vi "Calcul centroid.vi"(7 "Data PID":refnum<queue>, 8 "error in (no error)":errorcluster caption="entrée d'erreur (pas d'erreur)", 9 "Activer PID":bool, 10 "ROI":i16[][](array[numeric]), 11 "Data Cam Processing":T1 {"sigma X" format="%0.2f"; "mean X" format="%0.2f"; "mean Y" format="%0.2f"; "sigma Y" format="%0.2f"; "Shutter (us)" scale=22.0..10000000.0; "Gain Caméra" scale=0.0..1023.0}) -> (0 "error out":errorcluster caption="sortie d'erreur", 1 "CY brut":dbl, 2 "CX brut":dbl, 3 "Data Cam Processing 2":T1 {"sigma X" format="%0.2f"; "mean X" format="%0.2f"; "mean Y" format="%0.2f"; "sigma Y" format="%0.2f"; "Shutter (us)" scale=22.0..10000000.0; "Gain Caméra" scale=0.0..1023.0})   [LabVIEW 2026]
uses:
  Data-Processing.ctl
  <vilib>/Serenial/G Industrial Camera/g_industrial_cam/Buffer/Buffer.lvclass
  <vilib>/Serenial/G Industrial Camera/g_industrial_cam/Camera/Camera.lvclass
  <vilib>/picture/picture.llb/imagedata.ctl
  Data PID.ctl
  Etat_PID.ctl
  Set CX_CY.ctl
  <vilib>/ptbypt/NI_PtbyPt.lvlib
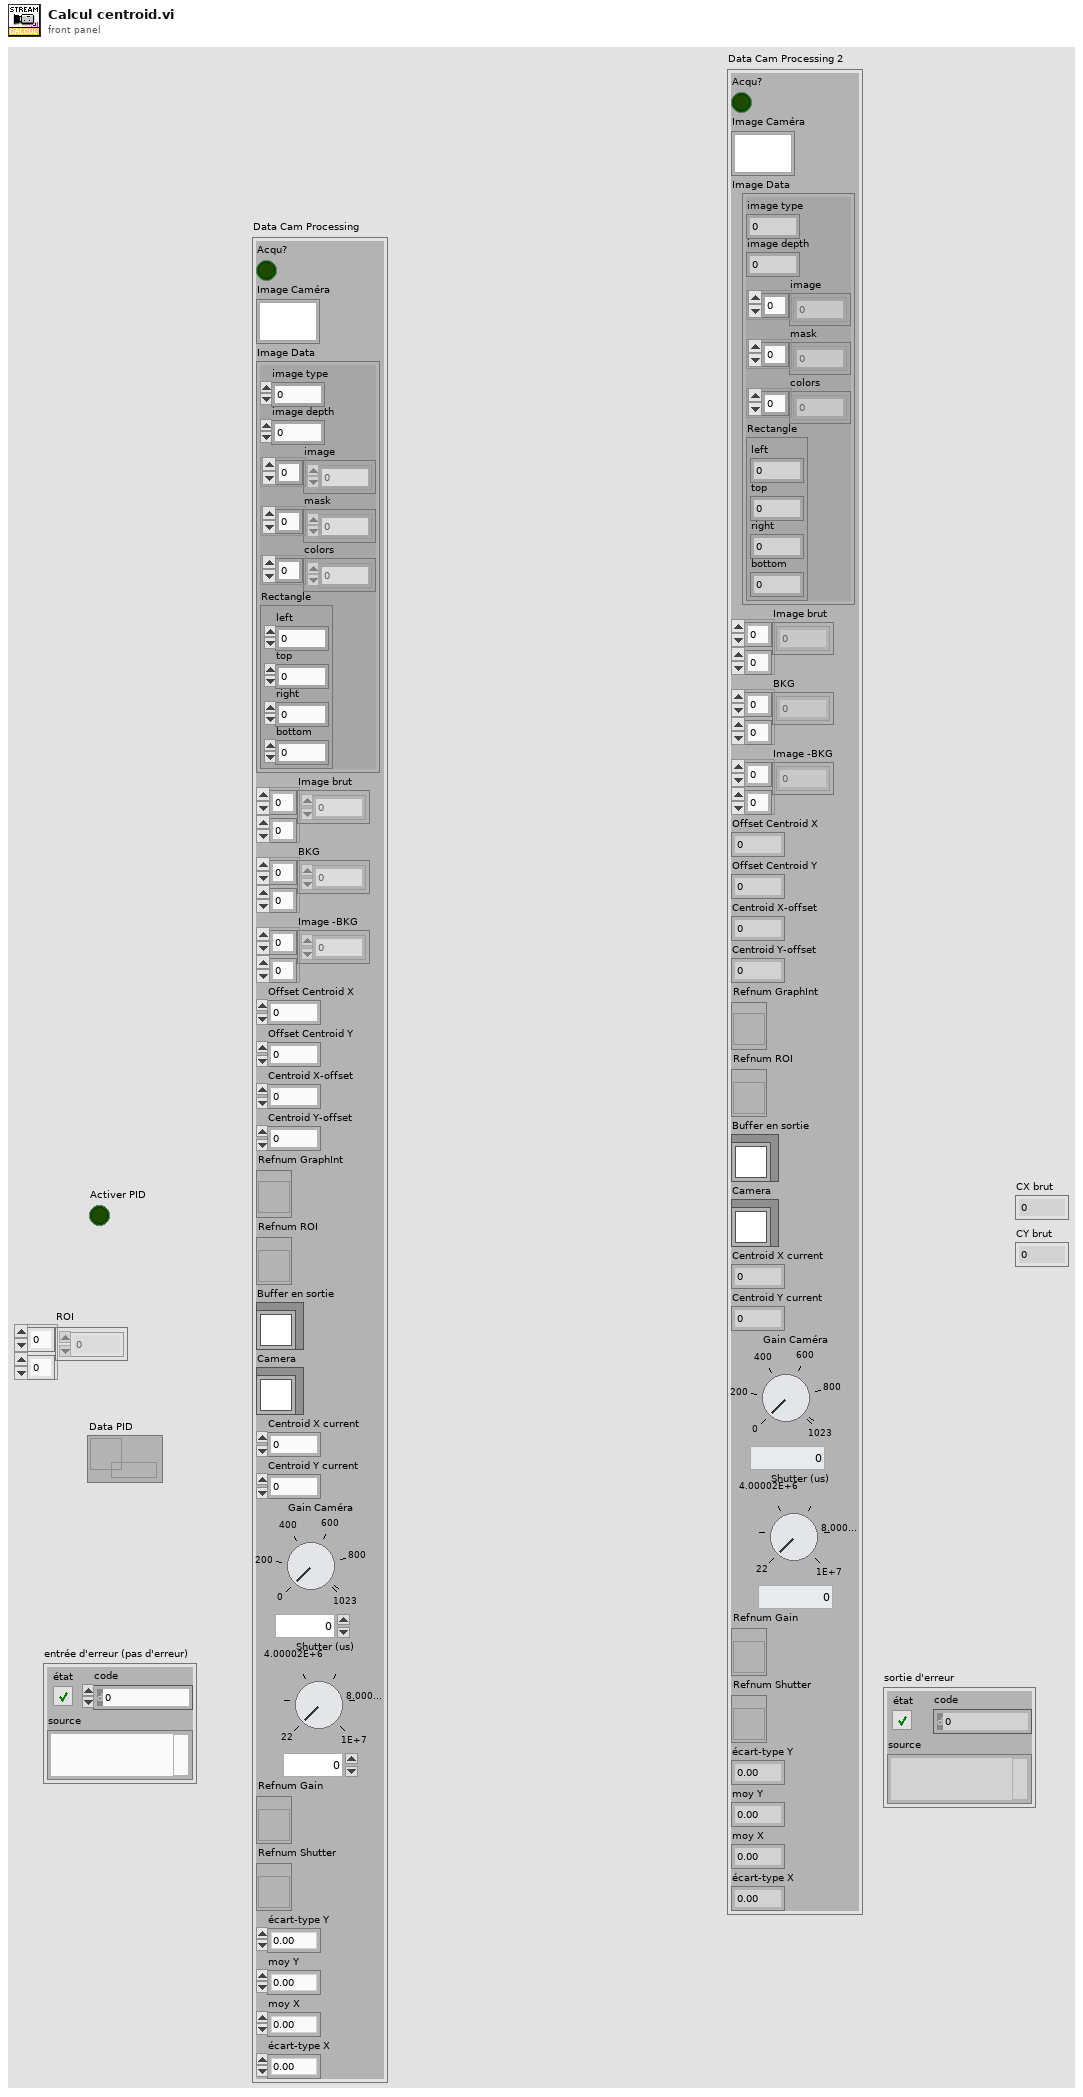
[diagram p1: front panel]
types:
  T1 = typedef "Data-Processing.ctl" = cluster{"Acqu?":bool, "Image Caméra":picture, "Image Data":T2, "Image brut":i16[][], "BKG":i16[][], "Image -BKG":i16[][], "Offset Centroid X":dbl, "Offset Centroid Y":dbl, "Centroid X-offset":dbl, "Centroid Y-offset":dbl, "Refnum GraphInt":refnum<vi>, "Refnum ROI":refnum<vi>, "Buffer en sortie":refnum<class "Buffer.lvclass">, "Camera":refnum<class "Camera.lvclass">, "Centroid X current":dbl, "Centroid Y current":dbl, "Gain Caméra":i32, "Shutter (us)":dbl, "Refnum Gain":refnum<vi>, "Refnum Shutter":refnum<vi>, "sigma Y":dbl, "mean Y":dbl, "mean X":dbl, "sigma X":dbl}
  T2 = typedef "imagedata.ctl" = cluster{"image type":i32, "image depth":i32, "image":u8[], "mask":u8[], "colors":u32[], "Rectangle":cluster{"left":i16, "top":i16, "right":i16, "bottom":i16}}
  T3 = typedef "Set CX_CY.ctl" = cluster{"CX":dbl, "CY":dbl}
  T4 = typedef "Etat_PID.ctl" = enum16{"PID", "Stop", "Reset PID", "Set Centroid", "Set T-Cube"}
  T5 = typedef "Data PID.ctl" = cluster{"Etat PID":T4, "Data PID":variant}
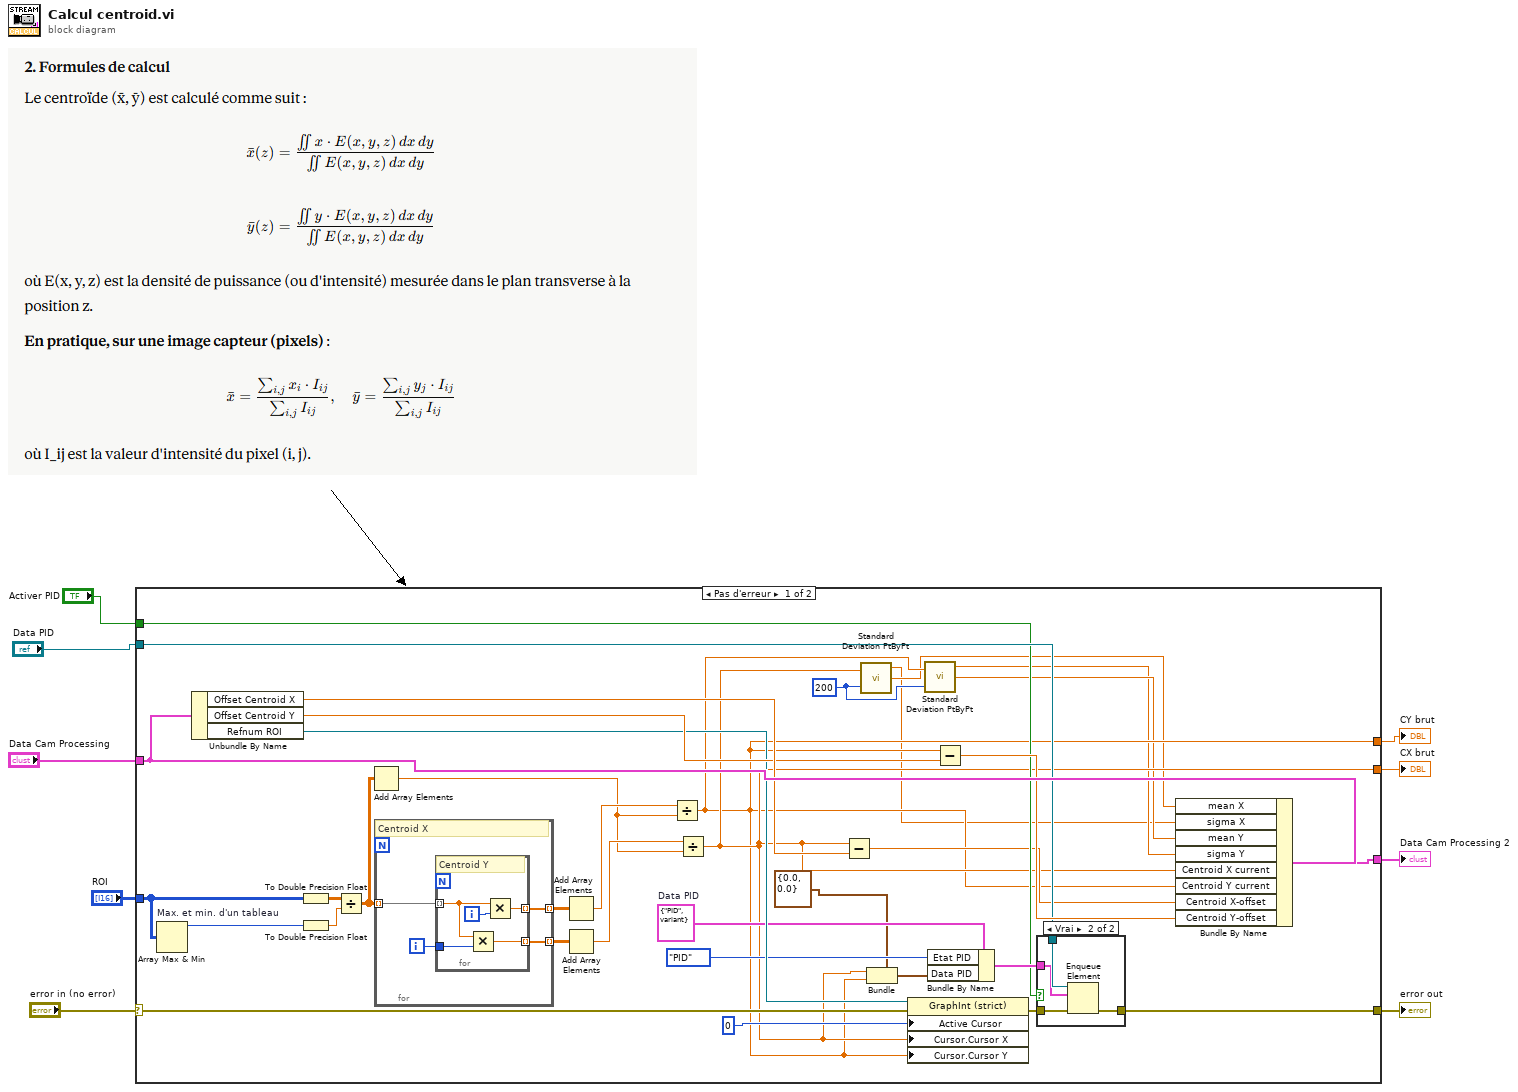
[diagram p0: block diagram]
diagram:
  n1 = case shown="Pas d'erreur" "error in (no error)" {
    selector: "error in (no error)" -> [w29 w60]
    tunnel: "ROI" -> [w38 _]
    tunnel: [w25 w60] -> w7
    tunnel: [w31 w59] -> w6
    tunnel: "Data Cam Processing" -> [w34 w59]
    tunnel: [w15 _] -> w4
    tunnel: [w14 _] -> w3
    tunnel: "Data PID" -> [w24 _]
    tunnel: "Activer PID" -> [w20 _]
    frame No Error {
      w16 = 200 ("sample length")
      w22 = T5 {"Etat PID"=enum."PID", "Data PID"=variant}  # Data PID
      n2 = Array Max & Min "Max. et min. d'un tableau"(array=w38) -> (max value=w39:i16)  [unwired: 3 out]
      n3 = Unbundle By Name(w34) -> ("Offset Centroid X"=w33:dbl, "Offset Centroid Y"=w32:dbl, "Refnum ROI"=w28:refnum<vi>)
      n4 = To Double Precision Float(number=w38) -> (double precision float=w36:dbl[][])
      n5 = To Double Precision Float(number=w39) -> (double precision float=w35:dbl)
      n6 = Divide(x=w36, y=w35) -> (x/y=w37:dbl[][])
      n7 = Add Array Elements(numeric array=w37) -> (sum=w40:dbl)
      n8 = for {
        tunnel: w37 -> [w52] mode=indexing
        tunnel: [w51] -> w44 mode=indexing
        tunnel: [w50] -> w42 mode=indexing
        i -> [w53]
        # "Centroid X"
        n9 = for {
          tunnel: w53 -> [w58]
          tunnel: w52 -> [w54] mode=indexing
          tunnel: [w57] -> w51 mode=indexing
          tunnel: [w55] -> w50 mode=indexing
          i -> [w56]
          # "Centroid Y"
          n10 = Multiply(x=w54, y=w58) -> (x*y=w57:dbl)
          n11 = Multiply(x=w54, y=w56) -> (x*y=w55:dbl)
        }
      }
      n12 = Add Array Elements(numeric array=w42) -> (sum=w41:dbl)
      n13 = Add Array Elements(numeric array=w44) -> (sum=w43:dbl)
      n14 = Divide(x=w41, y=w40) -> (x/y=w14:dbl)
      n15 = Divide(x=w43, y=w40) -> (x/y=w15:dbl)
      n16 = Subtract(x=w15, y=w33) -> (x-y=w19:dbl)
      n17 = call <vilib>:"Standard Deviation PtByPt.vi"("x"=w15, "sample length"=w16) -> ("standard deviation"=w10:dbl, "mean"=w11:dbl)  [unwired: 1 in, 1 out]
      n18 = Bundle(cluster=T3 {"CX"=0.0, "CY"=0.0}, "CX"=w15, "CY"=w14) -> (w18:T3)
      n19 = property on="Nœud de propriété" class="GraphInt (strict)"(reference=w28, error in=w29, "Active Cursor"=u32 0 ("Curseur actif"), "Cursor.Cursor X"=w15, "Cursor.Cursor Y"=w14) -> (error out=w26:errorcluster)  [unwired: 1 out]
      n20 = call <vilib>:"Standard Deviation PtByPt.vi"("x"=w14, "sample length"=w16) -> ("standard deviation"=w12:dbl, "mean"=w13:dbl)  [unwired: 1 in, 1 out]
      n21 = Bundle By Name(cluster=w22, "Etat PID"=Etat_PID."PID", "Data PID"=w18) -> (w21:T5)
      n22 = Subtract(x=w14, y=w32) -> (x-y=w27:dbl)
      n23 = case shown="Vrai" w20 {
        tunnel: w26 -> [w45 w49]
        tunnel: [w45 w48] -> w25
        tunnel: w24 -> [_ w47]
        tunnel: w21 -> [_ w46]
        frame False {
        }
        frame True {
          n24 = Enqueue Element(queue=w47, element=w46, error in (no error)=w49) -> (error out=w48:errorcluster)  [unwired: 1 in, 2 out]
        }
      }
      n25 = Bundle By Name(cluster=w34, "mean X"=w11, "sigma X"=w10, "mean Y"=w13, "sigma Y"=w12, "Centroid X current"=w15, "Centroid Y current"=w14, "Centroid X-offset"=w19, "Centroid Y-offset"=w27) -> (w31:T1)
    }
    frame Error {
    }
  }
  "error out" <- w7
  "Data Cam Processing 2" <- w6
  "CX brut" <- w4
  "CY brut" <- w3
